vi "Подзавод2.vi"(9 "milliseconds to wait":u32, 10 "Хранилище in":T1, 11 "Количество":dbl) -> (3 "Хранилище out":T1)   [LabVIEW 2021]
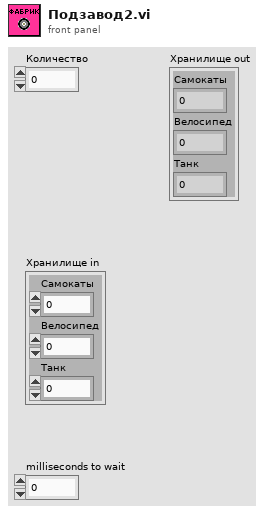
[diagram p1: front panel]
types:
  T1 = cluster{"Самокаты":dbl, "Велосипед":dbl, "Танк":dbl}
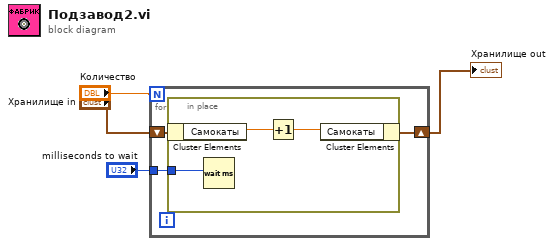
[diagram p0: block diagram]
diagram:
  n1 = for {
    N: "Количество" -> [_]
    shift-right: [w6] -> w2
    shift-left: "Хранилище in" -> [w7]
    tunnel: "milliseconds to wait" -> [w5]
    n2 = in-place {
      in-place-border: w5 -> [w8]
      n3 = in-place-cluster #1(w7) -> ("Самокаты"=w10:dbl)
      n4 = Wait (ms)(milliseconds to wait=w8) -> ()  [unwired: 1 out]
      n5 = Increment(x=w10) -> (x+1=w9:dbl)
      n6 = in-place-cluster #1("Самокаты"=w9) -> (w6:T1)
    }
  }
  "Хранилище out" <- w2
